vi "FPGA_init_single_scan.vi"(2 "error in":errorcluster, 3 "data":T1) -> (0 "error out":errorcluster)   [LabVIEW 2015]
uses:
  <vilib>/FPGAPlugInAG/PCIe-7841R/niLvFpga_Open_PCIe-7841R.vi
  <vilib>/rvi/interface/common/dynamic/niFpgaDynamicAddResources.vi
  <vilib>/Utility/error.llb/Error Cluster From Error Code.vi
  <vilib>/rvi/errors/niLvFpgaAdjustHostInterfaceError.vi
  <vilib>/FPGAPlugInAG/Dynamic/niLvFpga_Run_Dynamic.vi
  <vilib>/FPGAPlugInAG/Dynamic/niLvFpga_Close_Dynamic.vi
  GLOBAL/Global_FPGA.vi
  <vilib>/rvi/interface/nirviOpenFPGA/nirviOpenFPGA.xnode
  FPGA/FPGA Bitfiles/FPGAv0_FPGATarget_FPGAtriggercamer_8mvrEZH3eNo.lvbitx
  <vilib>/rvi/interface/nirviReadWriteControl/nirviReadWriteControl.xnode
  <vilib>/rvi/interface/nirviMethod/nirviMethod.xnode
  <vilib>/rvi/interface/nirviCloseFPGA/nirviCloseFPGA.xnode
  NiFpgaLv.dll
  <vilib>/rvi/interface/Simulation/niFpgaSimulationCallBeginRW.vi
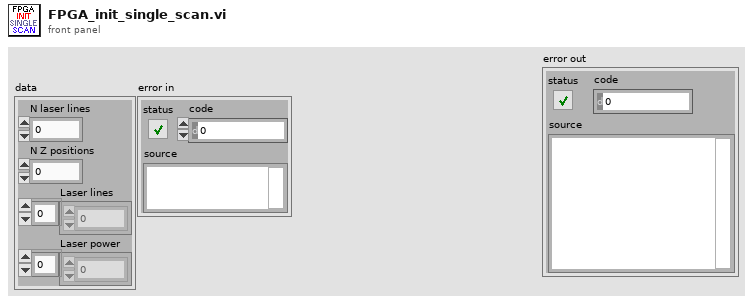
[diagram p1: front panel]
types:
  T1 = cluster{"N laser lines":i32, "N Z positions":i32, "Laser lines":i32[], "Laser power":sgl[]}
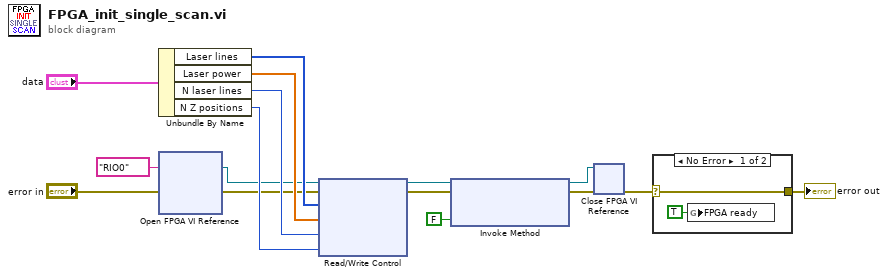
[diagram p0: block diagram]
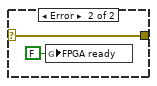
[diagram p2: hidden frame]
diagram:
  n1 = Unbundle By Name("data") -> ("Laser lines"=w10:i32[], "Laser power"=w11:sgl[], "N laser lines"=w12:i32, "N Z positions"=w13:i32)
  n2 = xnode "Open FPGA VI Reference"("error in"="error in", "resource name"=tag "RIO0") -> ("FPGA VI Reference Out"=w6:refnum<k20>, "error out"=w5:errorcluster)
  n3 = xnode "Read/Write Control"("FPGA VI Reference In"=w6, "error in"=w5, "Laser lines"=w10, "Laser power"=w11, "N laser lines"=w12, "N Z positions"=w13) -> ("FPGA VI Reference Out"=w7:refnum<k20>, "error out"=w8:errorcluster)
  n4 = xnode "Invoke Method"("FPGA VI Reference In"=w7, "error in"=w8, "Wait Until Done (F)"=FALSE) -> ("FPGA VI Reference Out"=w16:refnum<k20>, "error out"=w14:errorcluster)
  n5 = xnode "Close FPGA VI Reference"("FPGA VI Reference In"=w16, "error in"=w14) -> ("error out"=w15:errorcluster)
  n6 = case shown="No Error" w15 {
    selector: w15 -> [w17 w19]
    tunnel: [w17 w19] -> w1
    frame No Error {
      n7 = global write "Global_FPGA.vi" "FPGA ready"(TRUE ("FPGA ready")) -> ()
    }
    frame Error {
      n8 = global write "Global_FPGA.vi" "FPGA ready"(FALSE ("FPGA ready")) -> ()
    }
  }
  "error out" <- w1
